vi "CreateStopEvent.vi"(8 "error in (no error)":errorcluster, 11 "TCP_serverGUI in":refnum<class "TCP_serverGUI.lvclass">) -> (0 "error out":errorcluster, 2 "Event Registration Refnum":refnum<event-registration>, 3 "TCP_serverGUI out":refnum<class "TCP_serverGUI.lvclass">)   [LabVIEW 2023, in "TCP_serverGUI.lvlib" / "TCP_serverGUI.lvclass"]
uses:
  TCP_serverGUI.lvclass
  TypeDefinitions/CustomEvents.ctl
  TCP_serverGUI.lvclass/TCP_serverGUI.ctl
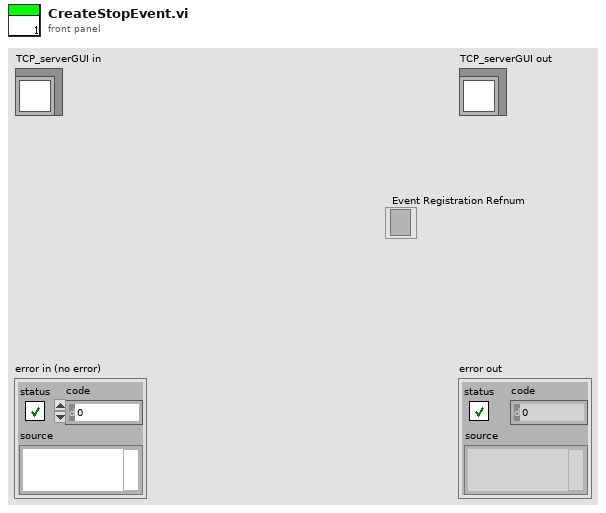
[diagram p1: front panel]
types:
  T1 = typedef "TCP_serverGUI.lvlib/TCP_serverGUI.lvclass/CustomEvents.ctl" = cluster{"Stop":refnum<user-event>}
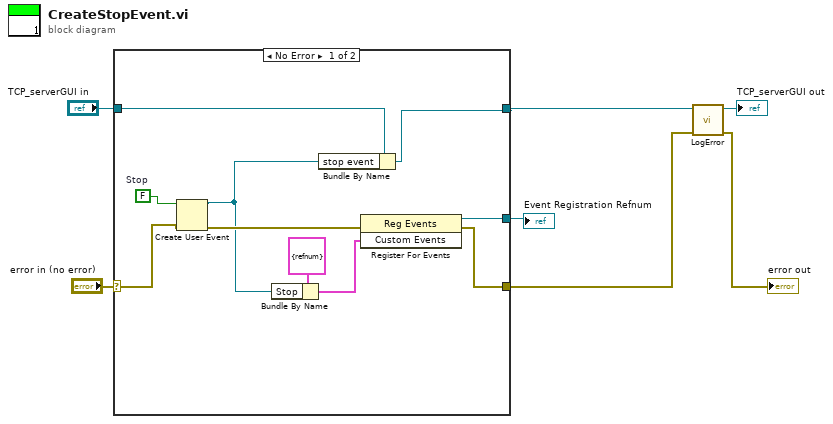
[diagram p0: block diagram]
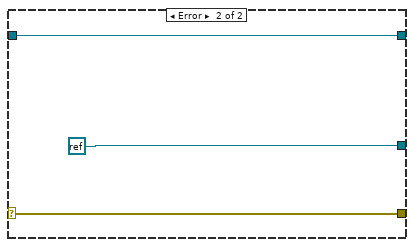
[diagram p2: hidden frame]
diagram:
  n1 = case shown="No Error" "error in (no error)" {
    selector: "error in (no error)" -> [w16 w20]
    tunnel: [w12 w20] -> w2
    tunnel: [w14 w19] -> w4
    tunnel: "TCP_serverGUI in" -> [w15 w19]
    tunnel: [w8 refnum<k0> refnum] -> w5
    frame No Error {
      w17 = FALSE  # Stop
      n2 = Create User Event(user event datatype=w17, error in=w16) -> (user event=w11:refnum<user-event>, error out=w13:errorcluster)
      n3 = Bundle By Name(cluster=T1 {"Stop"=refnum} ("Custom Events"), "Stop"=w11) -> (w10:T1)
      n4 = Bundle By Name(cluster=w15, "stop event"=w11) -> (w14:refnum<class "TCP_serverGUI.lvclass">)
      n5 = register-events(error in=w13, w10) -> (reference out=w8:refnum<event-registration>, error out=w12:errorcluster)  [unwired: 1 in]
    }
    frame Error {
    }
  }
  "Event Registration Refnum" <- w5
  n6 = call "LogError.vi"("error in (no error)"=w2, "TCP_serverGUI in"=w4) -> ("error out"=→"error out":errorcluster, "TCP_serverGUI out"=→"TCP_serverGUI out":refnum<class "TCP_serverGUI.lvclass">)  [unwired: 8 in]
